vi "Reset Calenda Value.vi"() -> ()   [LabVIEW 2010]
panel:
  out "错误输出":errorcluster
  out "Month":i16
  out "Day":i16
  in  "停止":bool
  in  "Calendar":refnum<k7>(container)
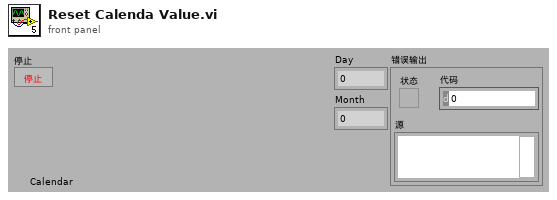
[diagram p1: front panel]
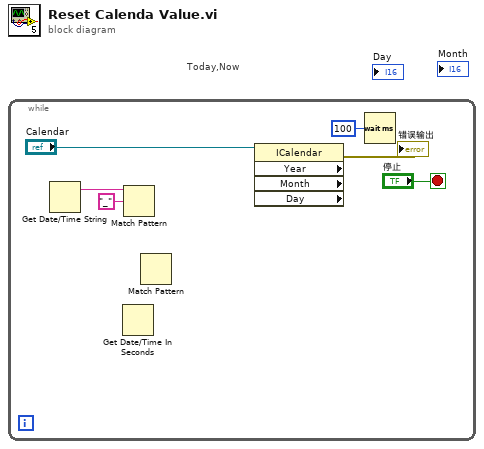
[diagram p0: block diagram]
diagram:
  # "Today,Now"
  n1 = while {
    stop <- "停止" stop-if-true
    n2 = Get Date/Time String() -> (date string=w2:string)  [unwired: 3 in, 1 out]
    n3 = Get Date/Time In Seconds() -> ()  [unwired: 1 out]
    n4 = Match Pattern(string=w2, regular expression="_" ("正则表达式")) -> ()  [unwired: 1 in, 4 out]
    n5 = Match Pattern() -> ()  [unwired: 3 in, 4 out]
    n6 = property class="ICalendar" props=["Year", "Month", "Day"](reference="Calendar") -> (error out=→"错误输出":errorcluster)  [unwired: 1 in, 4 out]
    n7 = Wait (ms)(milliseconds to wait=u32 100 ("等待时间（毫秒）")) -> ()  [unwired: 1 out]
  }
